vi "write_params.vi"(8 "error in (no error)":errorcluster, 10 "params":T1={"alpha"=1.0, "fit_prior"=TRUE, "class_prior"=[]}, 11 "MultinomialNB in":refnum<class "MultinomialNB.lvclass">) -> (0 "error out":errorcluster, 3 "MultinomialNB out":refnum<class "MultinomialNB.lvclass">)   [LabVIEW 2020, in "MultinomialNB.lvclass"]
uses:
  MultinomialNB.lvclass
  Controls/multinomial_nb_params.ctl
  MultinomialNB.lvclass/MultinomialNB.ctl
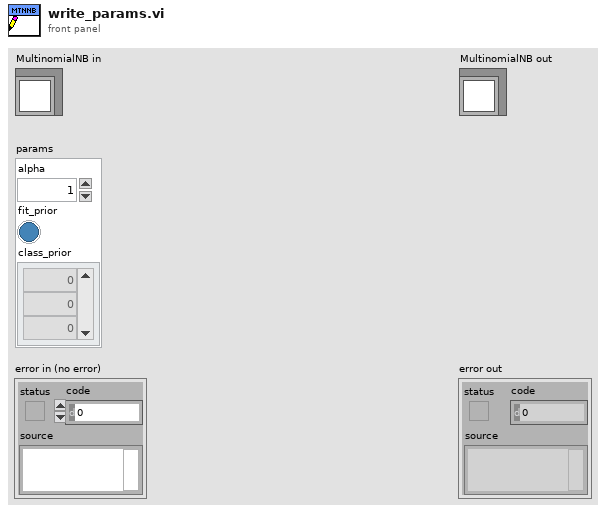
[diagram p1: front panel]
types:
  T1 = typedef "multinomial_nb_params.ctl" = cluster{"alpha":dbl, "fit_prior":bool, "class_prior":dbl[]}
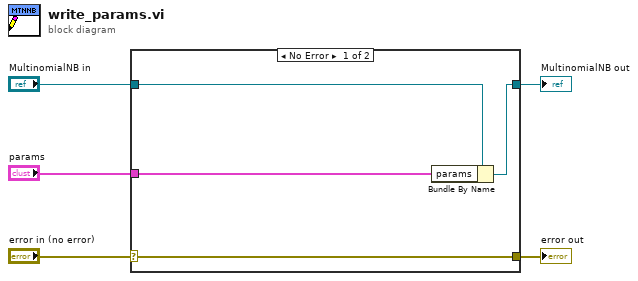
[diagram p0: block diagram]
diagram:
  n1 = case shown="No Error" "error in (no error)" {
    selector: "error in (no error)" -> [w9 w10]
    tunnel: [w9 w10] -> w4
    tunnel: [w7 w11] -> w2
    tunnel: "MultinomialNB in" -> [w8 w11]
    tunnel: "params" -> [w6 _]
    frame No Error {
      n2 = Bundle By Name(cluster=w8, "params"=w6) -> (w7:refnum<class "MultinomialNB.lvclass">)
    }
    frame Error {
    }
  }
  "error out" <- w4
  "MultinomialNB out" <- w2
